vi "Create JUnit Report.vi"(6 "Verbose":bool, 8 "error in (no error)":errorcluster, 10 "Report Path":path, 11 "Test Report.JUnit in":refnum<class "Test Report.JUnit.lvclass">) -> (0 "error out":errorcluster, 3 "Test Report.JUnit out":refnum<class "Test Report.JUnit.lvclass">)   [LabVIEW 2013, in "Caraya.lvlib" / "Test Report.JUnit.lvclass"]
uses:
  Test Report.JUnit.lvclass
  MsgSerializer.XML/MsgSerializer.XML.lvclass
  Test Report/Test Report.lvclass/Test Report.ctl
  Test Report/Test Report.lvclass
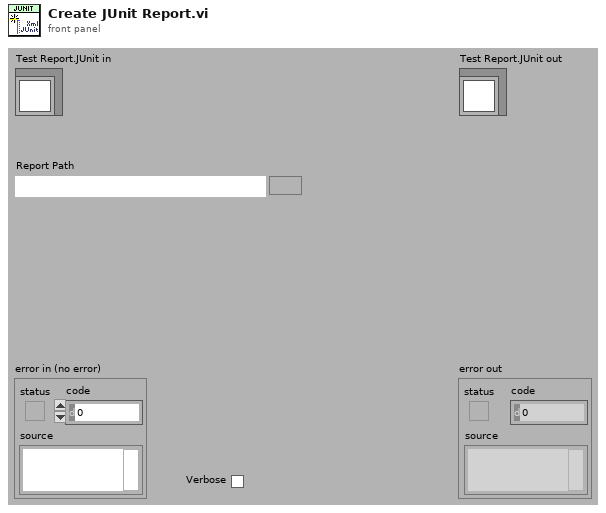
[diagram p1: front panel]
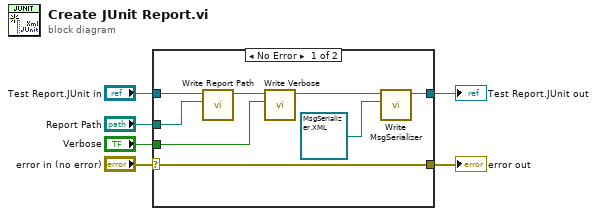
[diagram p0: block diagram]
diagram:
  n1 = case shown="No Error" "error in (no error)" {
    selector: "error in (no error)" -> [w14 w16]
    tunnel: [w14 w16] -> w5
    tunnel: [w8 w15] -> w3
    tunnel: "Test Report.JUnit in" -> [w13 w15]
    tunnel: "Report Path" -> [w12 _]
    tunnel: "Verbose" -> [w10 _]
    frame No Error {
      n2 = call "Write Report Path.vi"("Report Path"=w12, "Test Report.Default in"=w13) -> ("Test Report.Default out"=w11:refnum<class "Test Report.JUnit.lvclass">)  [unwired: 9 in]
      n3 = call "Write Verbose.vi"("Verbose"=w10, "Test Report in"=w11) -> ("Test Report out"=w9:refnum<class "Test Report.JUnit.lvclass">)  [unwired: 8 in, 1 out]
      n4 = call "Write MsgSerializer.vi"("MsgSerializer"=refnum<class "MsgSerializer.XML.lvclass"> refnum ("Caraya.lvlib:MsgSerializer.XMLProperty.lvclass"), "Test Report in"=w9) -> ("Test Report out"=w8:refnum<class "Test Report.JUnit.lvclass">)  [unwired: 9 in]
    }
    frame Error {
    }
  }
  "error out" <- w5
  "Test Report.JUnit out" <- w3
